vi "panel.SetOrigin.vi"(4 "error in":errorcluster, 5 "VIRef":refnum<vi> caption="VIRef ('caller' if not wired)") -> (0 "error out":errorcluster)   [LabVIEW 2020]
uses:
  <vilib>/Utility/miscctls.llb/LVPointTypeDef.ctl
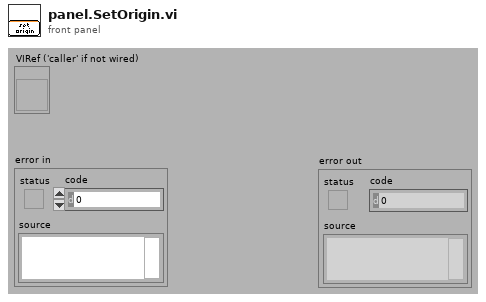
[diagram p1: front panel]
types:
  T1 = typedef "LVPointTypeDef.ctl" = cluster{"Horizontal":i16, "Vertical":i16}
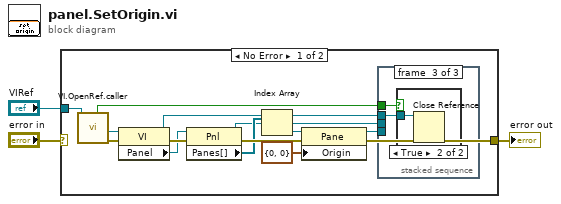
[diagram p0: block diagram]
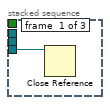
[diagram p2: hidden frame]
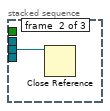
[diagram p3: hidden frame]
diagram:
  n1 = case shown="No Error" "error in" {
    selector: "error in" -> [_ w23]
    tunnel: [w12 w23] -> w3
    tunnel: "VIRef" -> [w9 _]
    frame No Error {
      n2 = call "VI.OpenRef.caller.vi"("VI.ref"=w9) -> ("error out"=w10:errorcluster, "VI.ref out"=w11:refnum<vi>, "opened new?"=w4:bool)  [unwired: 2 in, 6 out]
      n3 = property class="VI"(reference=w11, error in=w10) -> (reference out=w5:refnum<vi>, error out=w16:errorcluster, "Panel"=w13:refnum<vi>)
      n4 = property class="Pnl"(reference=w13, error in=w16) -> (reference out=w6:refnum<vi>, error out=w17:errorcluster, "Panes[]"=w14:refnum<vi>[])
      n5 = Index Array(array=w14) -> (element=w15:refnum<vi>)  [unwired: 1 in]
      n6 = property class="Pane"(reference=w15, error in=w17, "Origin"=T1 {"Horizontal"=0, "Vertical"=0}) -> (reference out=w7:refnum<vi>, error out=w12:errorcluster)
      n7 = stacked-sequence {
        tunnel: w7 -> [w18 _ _]
        tunnel: w6 -> [_ w19 _]
        tunnel: w5 -> [_ _ w21]
        tunnel: w4 -> [_ _ w20]
        frame #0 {
          n8 = Close Reference(reference=w18) -> ()  [unwired: 1 in, 1 out]
        }
        frame #1 {
          n9 = Close Reference(reference=w19) -> ()  [unwired: 1 in, 1 out]
        }
        frame #2 {
          n10 = case shown="True" w20 {
            tunnel: w21 -> [_ w22]
            frame False {
            }
            frame True {
              n11 = Close Reference(reference=w22) -> ()  [unwired: 1 in, 1 out]
            }
          }
        }
      }
    }
    frame Error {
    }
  }
  "error out" <- w3
